vi "Write Label at Path(Array).vi"(8 "error in (no error)":errorcluster, 9 "Name":string, 10 "Path in":string[](array[string]), 11 "Variant in":variant) -> (0 "error out":errorcluster, 3 "Variant out":variant)   [LabVIEW 2017, in "Variant Data Manipulation.lvlib"]
uses:
  Variant Data Manipulation.lvlib
  <vilib>/Utility/Data Type/NI_Data Type.lvlib
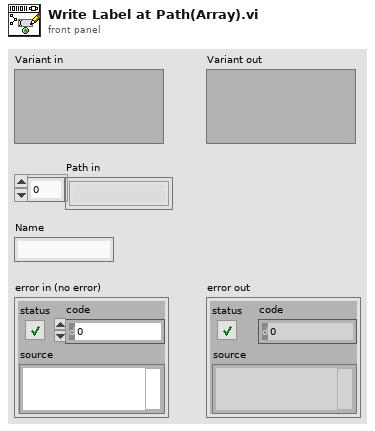
[diagram p1: front panel]
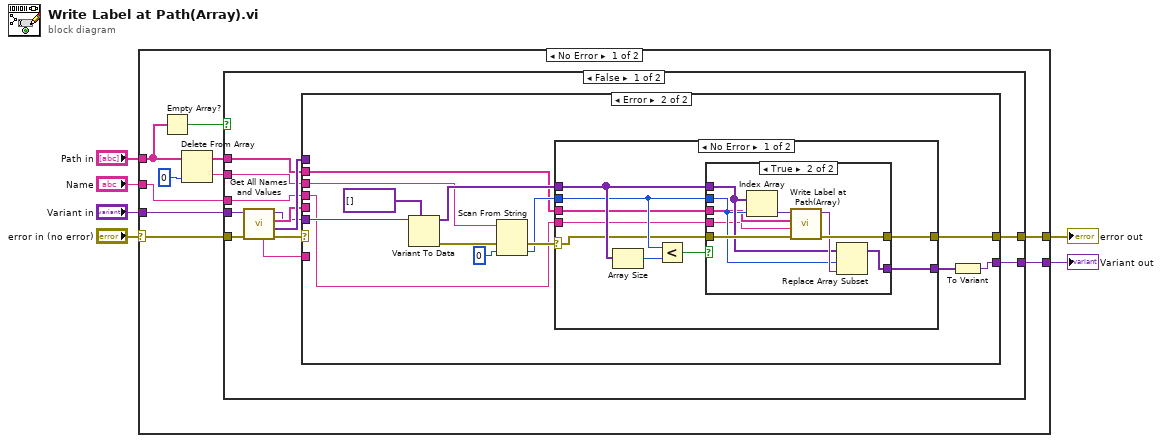
[diagram p0: block diagram]
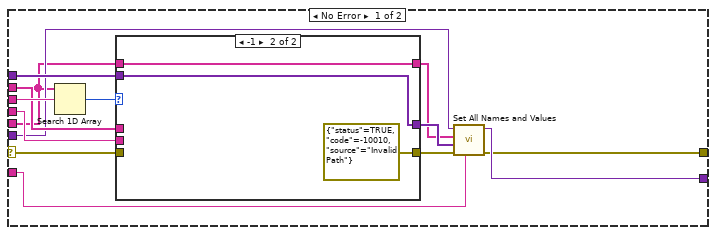
[diagram p2: hidden frame]
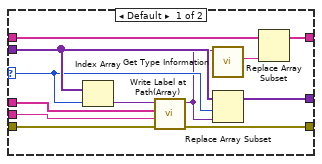
[diagram p3: hidden frame]
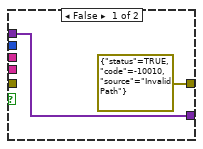
[diagram p4: hidden frame]
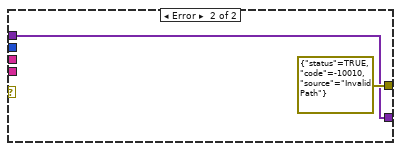
[diagram p5: hidden frame]
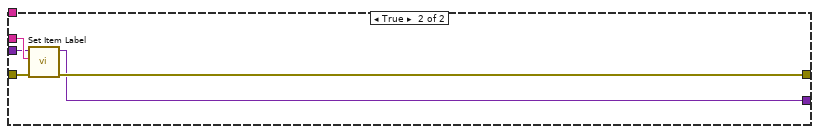
[diagram p6: hidden frame]
diagram:
  n1 = case shown="No Error" "error in (no error)" {
    selector: "error in (no error)" -> [w15 w99]
    tunnel: "Path in" -> [w7 _]
    tunnel: "Variant in" -> [w16 w98]
    tunnel: [w9 w99] -> w4
    tunnel: [w10 w98] -> w2
    tunnel: "Name" -> [w11 _]
    frame No Error {
      n2 = Empty Array?(array=w7) -> (empty?=w12:bool)
      n3 = Delete From Array(array=w7, index=0) -> (deleted portion=w14:string, array with subset deleted=w8:string[])  [unwired: 1 in]
      n4 = case shown="False" w12 {
        tunnel: w16 -> [w28 w93]
        tunnel: w15 -> [w27 w97]
        tunnel: w14 -> [w24 _]
        tunnel: w8 -> [w23 _]
        tunnel: w11 -> [w22 w94]
        tunnel: [w18 w95] -> w10
        tunnel: [w17 w96] -> w9
        frame False {
          n5 = call "Get All Names and Values.vi"("error in"=w27, "Cluster in"=w28) -> ("error out"=w26:errorcluster, "Values"=w25:variant[], "Element Names"=w21:string[], "Cluster out"=w20:variant, "Cluster Name"=w19:string)  [unwired: 5 in]
          n6 = case shown="Error" w26 {
            selector: w26 -> [w40 _]
            tunnel: w20 -> [w31 w67]
            tunnel: w24 -> [w39 w58]
            tunnel: w21 -> [w30 _]
            tunnel: w25 -> [w41 _]
            tunnel: w23 -> [w38 w62]
            tunnel: w22 -> [w37 w63]
            tunnel: w19 -> [w36 _]
            tunnel: [w33 w61] -> w18
            tunnel: [w32 w59] -> w17
            frame No Error {
              n7 = Search 1D Array(1D array=w30, element=w39) -> (index of element=w42:i32)  [unwired: 1 in]
              n8 = case shown="-1" w42 {
                selector: w42 -> [w50 _]
                tunnel: [w52 errorcluster {"status"=TRUE, "code"=-10010, "source"="Invalid Path"} ("error IO")] -> w34
                tunnel: w41 -> [w51 w56]
                tunnel: w40 -> [w53 _]
                tunnel: w38 -> [w48 _]
                tunnel: w37 -> [w47 _]
                tunnel: [w49 w56] -> w35
                tunnel: w30 -> [w44 w55]
                tunnel: [w43 w55] -> w29
                frame Default {
                  n9 = Index Array(array=w51, index=w50) -> (element=w54:variant)
                  n10 = call "Write Label at Path(Array).vi"("error in (no error)"=w53, "Name"=w47, "Path in"=w48, "Variant in"=w54) -> ("error out"=w52:errorcluster, "Variant out"=w46:variant)  [unwired: 6 in]
                  n11 = call <vilib>:"Get Type Information.vi"("Variant"=w46) -> ("Name"=w45:string)  [unwired: 6 in, 4 out]
                  n12 = Replace Array Subset(array=w51, new element=w46, index=w50) -> (w49:variant[])
                  n13 = Replace Array Subset(array=w44, new element=w45) -> (w43:string[])  [unwired: 1 in]
                }
                frame -1 {
                }
              }
              n14 = call "Set All Names and Values.vi"("Cluster Name"=w36, "error in"=w34, "values"=w35, "Element Names"=w29, "Cluster in"=w31) -> ("error out"=w32:errorcluster, "Cluster out"=w33:variant)  [unwired: 5 in]
            }
            frame Error {
              n15 = Variant To Data(type=variant[] [], Variant=w67) -> (data=w65:variant[], error out=w64:errorcluster)  [unwired: 1 in]
              n16 = Scan From String(input string=w58, error in=w64, default 1=0 ("default value 1")) -> (error out=w69:errorcluster, output 1=w68:i32)  [unwired: 2 in, 2 out]
              n17 = case shown="No Error" w69 {
                selector: w69 -> [w73 _]
                tunnel: [w74 errorcluster {"status"=TRUE, "code"=-10010, "source"="Invalid Path"} ("error IO")] -> w59
                tunnel: w68 -> [w77 _]
                tunnel: w65 -> [w78 w91]
                tunnel: [w79 w91] -> w60
                tunnel: w63 -> [w72 _]
                tunnel: w62 -> [w71 _]
                frame No Error {
                  n18 = Array Size(array=w78) -> (size(s)=w76:i32)
                  n19 = Less?(x=w77, y=w76) -> (x < y?=w75:bool)
                  n20 = case shown="True" w75 {
                    tunnel: [w80 w87] -> w79
                    tunnel: w78 -> [w80 w85]
                    tunnel: w77 -> [_ w84]
                    tunnel: [errorcluster {"status"=TRUE, "code"=-10010, "source"="Invalid Path"} ("error IO") w88] -> w74
                    tunnel: w73 -> [_ w89]
                    tunnel: w72 -> [_ w82]
                    tunnel: w71 -> [_ w83]
                    frame False {
                    }
                    frame True {
                      n21 = Index Array(array=w85, index=w84) -> (element=w90:variant)
                      n22 = call "Write Label at Path(Array).vi"("error in (no error)"=w89, "Name"=w82, "Path in"=w83, "Variant in"=w90) -> ("error out"=w88:errorcluster, "Variant out"=w86:variant)  [unwired: 6 in]
                      n23 = Replace Array Subset(array=w85, new element=w86, index=w84) -> (w87:variant[])
                    }
                  }
                }
                frame Error {
                }
              }
              n24 = To Variant(anything=w60) -> (Variant=w61:variant)
            }
          }
        }
        frame True {
          n25 = call "Set Item Label.vi"("error in (no error)"=w97, "Name"=w94, "Variant in"=w93) -> ("error out"=w96:errorcluster, "Variant out"=w95:variant)  [unwired: 7 in]
        }
      }
    }
    frame Error {
    }
  }
  "error out" <- w4
  "Variant out" <- w2
